vi "Send batch.vi"(8 "error in (no error)":errorcluster, 9 "motor port":u16=5001, 10 "motor ip":string, 11 "instruction":string) -> (0 "error out":errorcluster, 1 "error":bool, 2 "ok":bool, 3 "response":string, 5 "response array":string[](array[string]))   [LabVIEW 2018]
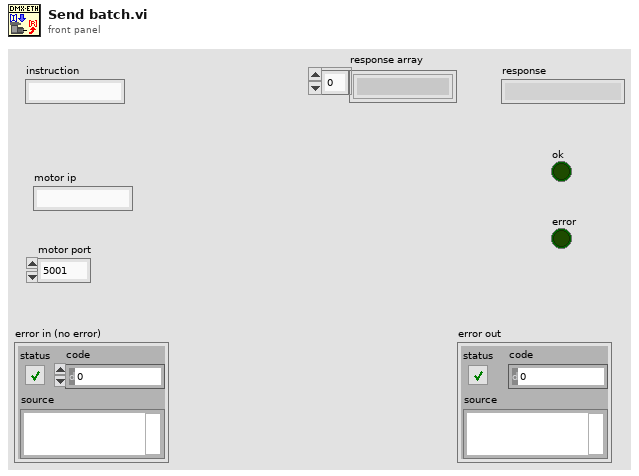
[diagram p1: front panel]
types:
  T1 = enum16{"Standard", "Buffered", "CRLF", "Immediate"}
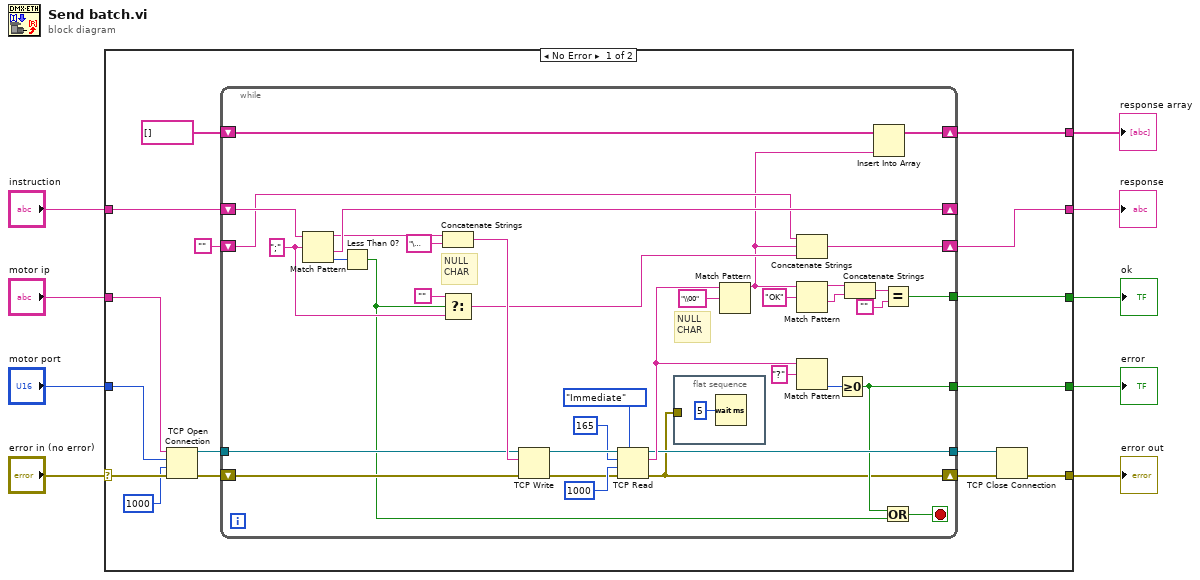
[diagram p0: block diagram]
diagram:
  n1 = case shown="No Error" "error in (no error)" {
    selector: "error in (no error)" -> [w19 w63]
    tunnel: [w16 w63] -> w9
    tunnel: [w22 _] -> w8
    tunnel: "instruction" -> [w23 _]
    tunnel: "motor ip" -> [w20 _]
    tunnel: "motor port" -> [w21 _]
    tunnel: [w25 _] -> w3
    tunnel: [w24 _] -> w2
    tunnel: [w10 _] -> w1
    frame No Error {
      n2 = TCP Open Connection(address=w20, remote port or service name=w21, timeout ms (60000)=1000, error in (no error)=w19) -> (connection ID=w15:refnum<k5>, error out=w18:errorcluster)  [unwired: 1 in]
      n3 = while {
        tunnel: [w52] -> w25
        tunnel: [w32] -> w24
        shift-right: [w26] -> w17
        shift-left: w18 -> [w35]
        shift-right: [w42] -> _
        shift-left: w23 -> [w44]
        shift-right: [w38] -> w22
        shift-left: "" -> [w30]
        tunnel: w15 -> [w36]
        tunnel: [w34] -> w14
        shift-right: [w28] -> w10
        shift-left: string[] [] ("response array") -> [w29]
        stop <- w33 stop-if-true
        w40 = ";" ("search string")
        # "NULL\nCHAR"
        # "NULL\nCHAR"
        n4 = Match Pattern(string=w44, regular expression=w40) -> (before substring=w41:string, after substring=w42:string, offset past match=w43:i32)  [unwired: 1 in, 1 out]
        n5 = Less Than 0?(x=w43) -> (x < 0?=w31:bool)
        n6 = Concatenate Strings(w41, "\u0000" ("search string")) -> (w51:string)
        n7 = Select(t="", s=w31, f=w40) -> (s? t:f=w37:string)
        n8 = TCP Write(connection ID=w36, data in=w51, error in (no error)=w35) -> (connection ID out=w61:refnum<k5>, error out=w49:errorcluster)  [unwired: 1 in, 1 out]
        n9 = TCP Read(connection ID=w61, bytes to read=165, error in (no error)=w49, 7:T1."Immediate" ("mode (standard)"), 9:1000 ("timeout ms (60000)")) -> (connection ID out=w34:refnum<k5>, data out=w47:string, error out=w26:errorcluster)
        n10 = flat-sequence {
          tunnel: w26 -> [_]
          frame #0 {
            n11 = Wait (ms)(milliseconds to wait=u32 5) -> ()  [unwired: 1 out]
          }
        }
        n12 = Match Pattern(string=w47, regular expression="\\00" ("search string")) -> (before substring=w27:string)  [unwired: 1 in, 3 out]
        n13 = Concatenate Strings(w30, w27, w37) -> (w38:string)
        n14 = Match Pattern(string=w27, regular expression="OK" ("y")) -> (before substring=w55:string, after substring=w48:string)  [unwired: 1 in, 2 out]
        n15 = Match Pattern(string=w47, regular expression="?") -> (offset past match=w45:i32)  [unwired: 1 in, 3 out]
        n16 = Greater Or Equal To 0?(x=w45) -> (x >= 0?=w32:bool)
        n17 = Concatenate Strings(w55, w48) -> (w54:string)
        n18 = Insert Into Array(array=w29, new element=w27) -> (w28:string[])  [unwired: 1 in]
        n19 = Equal?(x=w54, y="") -> (x = y?=w52:bool)
        n20 = Or(x=w32, y=w31) -> (x .or. y?=w33:bool)
      }
      n21 = TCP Close Connection(connection ID=w14, error in (no error)=w17) -> (error out=w16:errorcluster)  [unwired: 1 in, 1 out]
    }
    frame Error {
    }
  }
  "error out" <- w9
  "response" <- w8
  "ok" <- w3
  "error" <- w2
  "response array" <- w1
